vi "read_input_data.vi"(5 "Modulation info":T1={"Fs full"=0.0, "Fs high"=0.0, "Fs low"=0.0, "Read size"=5000, "FFT size low"=5000, "df low"=5000.0, "High carriers"=[], "Low carriers"=[], "Hi channels at low"=[7]} {"Hi channels at low" min=0 step=1; "Low carriers" format="%#_6p"; "High carriers" format="%#_6p"}, 7 "Config":T2={"IO params"={"Conversion"={"Rate"=4.0, "Num cards"=2, "Out channels"=4}, "Carriers"={"Phase shift"=180.0, "Levels"=[[0.8, 0.8, 0.8], [0.03, 0.03, 0.03]], "Delay samples"=73.15}, "TCP"={"Host"="192.168.1.15", "Port"=6666, "Buffering"=6, "Timeout"=6}, "Input channel sign"=[1, 1, 1]}, "High rate STFT"={"Win param"=101.5, "Window type"=61, "Win order"=2, "DFT size"=64, "Channels"=[7], "Oversample"=64}, "Low rate STFT"={"Win param"=120.0, "Window type"=61, "Win order"=8, "DFT size"=64, "Channels"=[7], "Oversample"=64}, "Filtering "=[]} {"Filtering"."Distortion"."Limit" format="%#_3p"; "Filtering"."Distortion"."LF cut" format="%#_3p"; "Filtering"."Kalman"."Measure noise" format="%#_3p"; "Filtering"."Kalman"."Process noise" format="%#_3p"; "Filtering"."Hum"."Limit" format="%#_3p"; "Filtering"."Hum"."Frequency" format="%#_4p"; "Low rate STFT"."Oversample" min=1 step=1; "Low rate STFT"."Channels" min=0 step=1; "Low rate STFT"."DFT size" min=1 step=1; "Low rate STFT"."Window type" items=["Rectangle"=0, "Hanning"=1, "Hamming"=2, "Blackman-Harris"=3, "Exact Blackman"=4, "Blackman"=5, "Flat Top"=6, "4 Term B-Harris "=7, "7 Term B-Harris"=8, "Low Sidelobe"=9, "Blackman Nuttall"=11, "Triangle"=30, "Bartlett-Hanning"=31, "Bohman"=32, "Parzen"=33, "Welch"=34, "Kaiser"=60, "Dolph-Chebyshev"=61, "Gaussian"=62]; "High rate STFT"."Oversample" min=1 step=1; "High rate STFT"."Channels" min=0 step=1; "High rate STFT"."DFT size" min=1 step=1; "High rate STFT"."Window type" items=["Rectangle"=0, "Hanning"=1, "Hamming"=2, "Blackman-Harris"=3, "Exact Blackman"=4, "Blackman"=5, "Flat Top"=6, "4 Term B-Harris "=7, "7 Term B-Harris"=8, "Low Sidelobe"=9, "Blackman Nuttall"=11, "Triangle"=30, "Bartlett-Hanning"=31, "Bohman"=32, "Parzen"=33, "Welch"=34, "Kaiser"=60, "Dolph-Chebyshev"=61, "Gaussian"=62]; "IO params"."Input channel sign" min=-1 max=1 step=1; "IO params"."Carriers"."Levels" min=0.0 step=0.1; "IO params"."Conversion"."Rate" format="%#_8g"}, 8 "error in":errorcluster, 11 "Connection in":refnum<k5>) -> (0 "error out":errorcluster, 1 "Restart IO":bool, 2 "Input data":waveform(dbl)[][](array[waveform]), 3 "Connection out":refnum<k5>, 4 "Sequence":u8)   [LabVIEW 2026]
uses:
  processing/ilemt_config.ctl
  IO_params.ctl
  processing/stft_params.ctl
  <vilib>/Analysis/4window.llb/windowTd.ctl
  processing/filter_params.ctl
  processing/detrend_mode.ctl
  processing/modulation_info.ctl
  <vilib>/Analysis/NI_AALPro.lvlib
panel:
  out "IO error":i32
  out "Sync error":i32
  out "length":i32
  in  "Timeouts":i32
  out "error IO":errorcluster
  # "Waveforms are scaled to range 0..1, rows are input cards and columns are XYZ channels."
  # "Read the input data using TCP"
  # "There was an error so we should restart IO"
  # "Locals:"
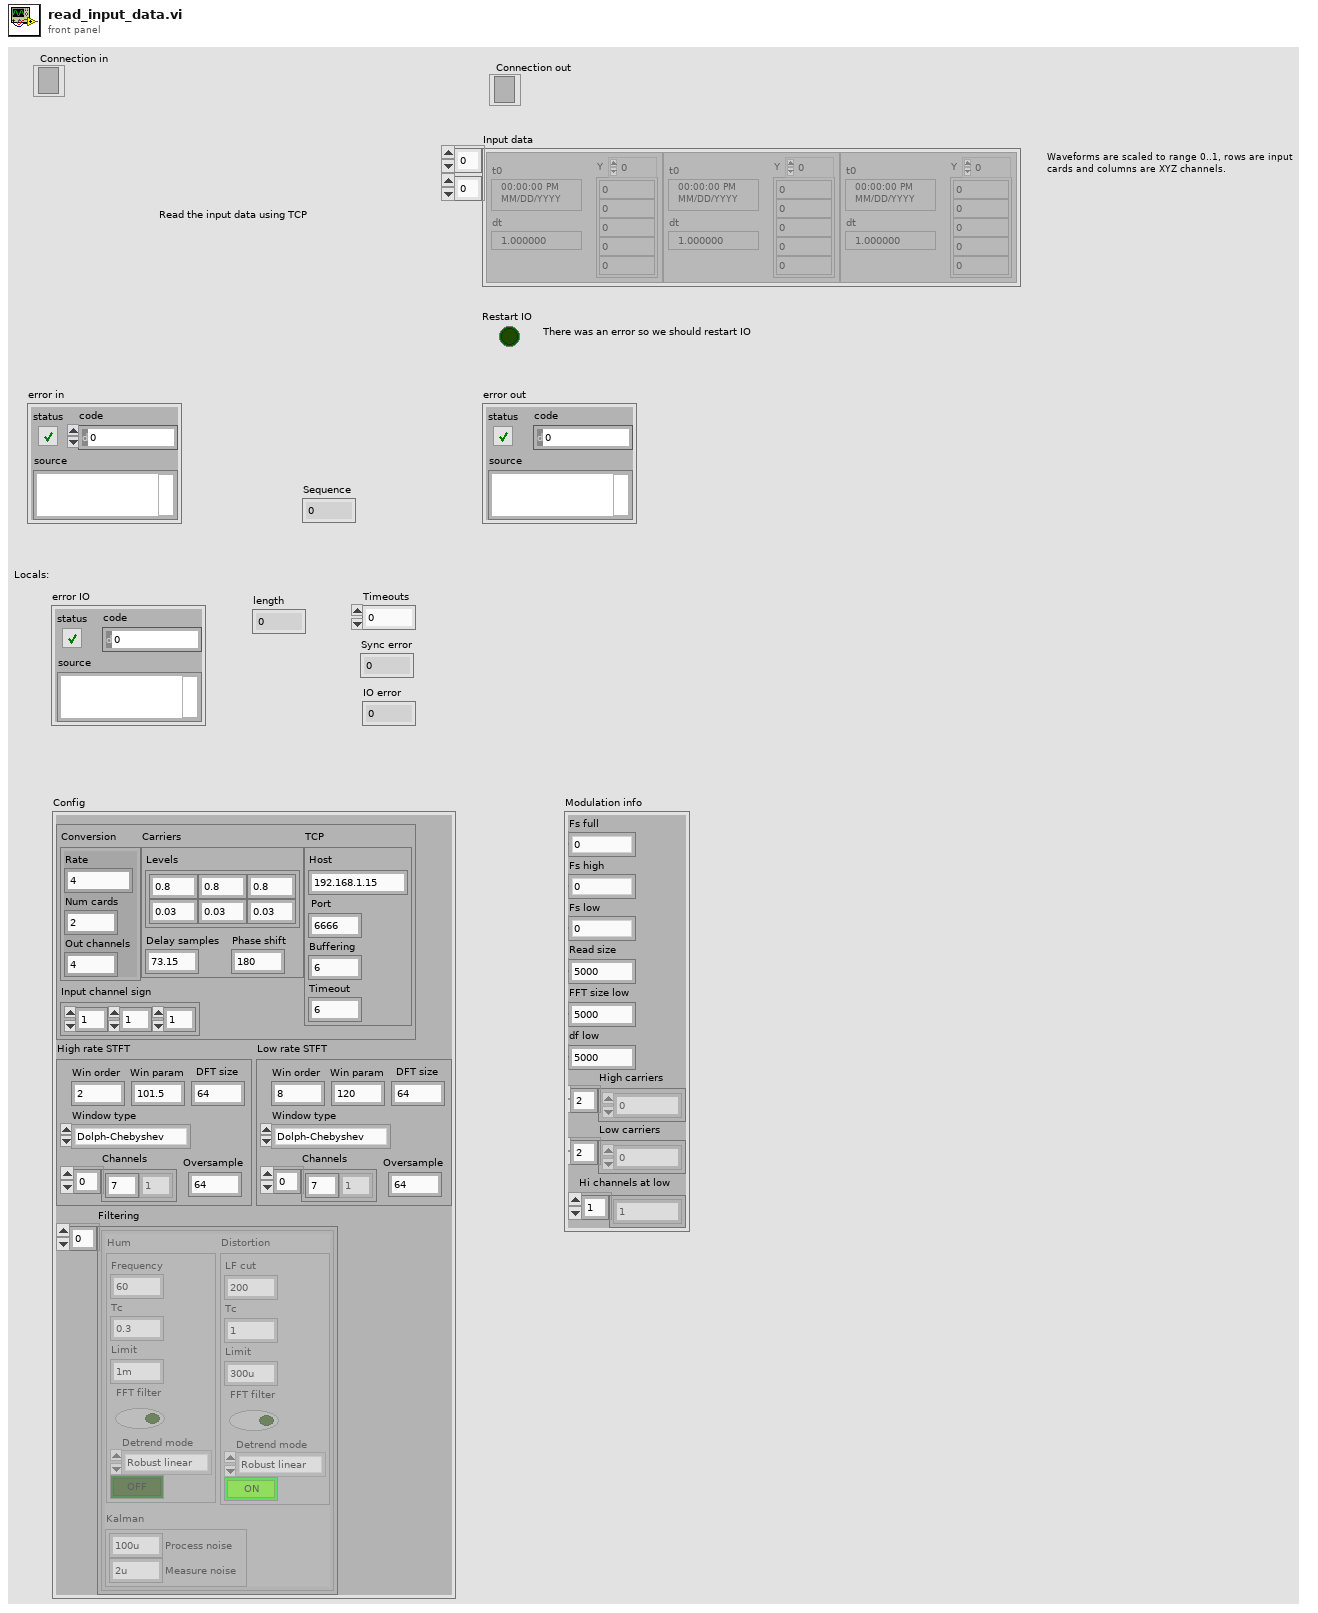
[diagram p1: front panel]
types:
  T1 = typedef "modulation_info.ctl" = cluster{"Fs full":dbl, "Fs high":dbl, "Fs low":dbl, "Read size":i32, "FFT size low":i32, "df low":dbl, "High carriers":dbl[], "Low carriers":dbl[], "Hi channels at low":i32[]}
  T2 = typedef "ilemt_config.ctl" = cluster{"IO params":T3, "High rate STFT":T4, "Low rate STFT":T4, "Filtering ":T6[]}
  T3 = typedef "IO_params.ctl" = cluster{"Conversion":cluster{"Rate":dbl, "Num cards":u32, "Out channels":u32}, "Carriers":cluster{"Phase shift":dbl, "Levels":dbl[][], "Delay samples":dbl}, "TCP":cluster{"Host":string, "Port":i32, "Buffering":u32, "Timeout":u32}, "Input channel sign":i32[]}
  T4 = typedef "stft_params.ctl" = cluster{"Win param":dbl, "Window type":T5, "Win order":i32, "DFT size":i32, "Channels":i32[], "Oversample":i32}
  T5 = typedef "NI_AALPro.lvlib/windowTd.ctl" = u32
  T6 = typedef "filter_params.ctl" = cluster{"Hum":cluster{"Frequency":dbl, "Tc":dbl, "Limit":dbl, "FFT filter":bool, "Detrend mode":T7, "Enable":bool}, "Kalman":cluster{"Process noise":dbl, "Measure noise":dbl}, "Distortion":cluster{"LF cut":dbl, "Tc":dbl, "Limit":dbl, "FFT filter":bool, "Detrend mode":T7, "Enable":bool}}
  T7 = typedef "detrend_mode.ctl" = enum16{"Zero mean", "Linear", "Robust linear"}
  T8 = enum16{"Standard", "Buffered", "CRLF", "Immediate"}
  T9 = enum16{"big-endian, network order", "native, host order", "little-endian"}
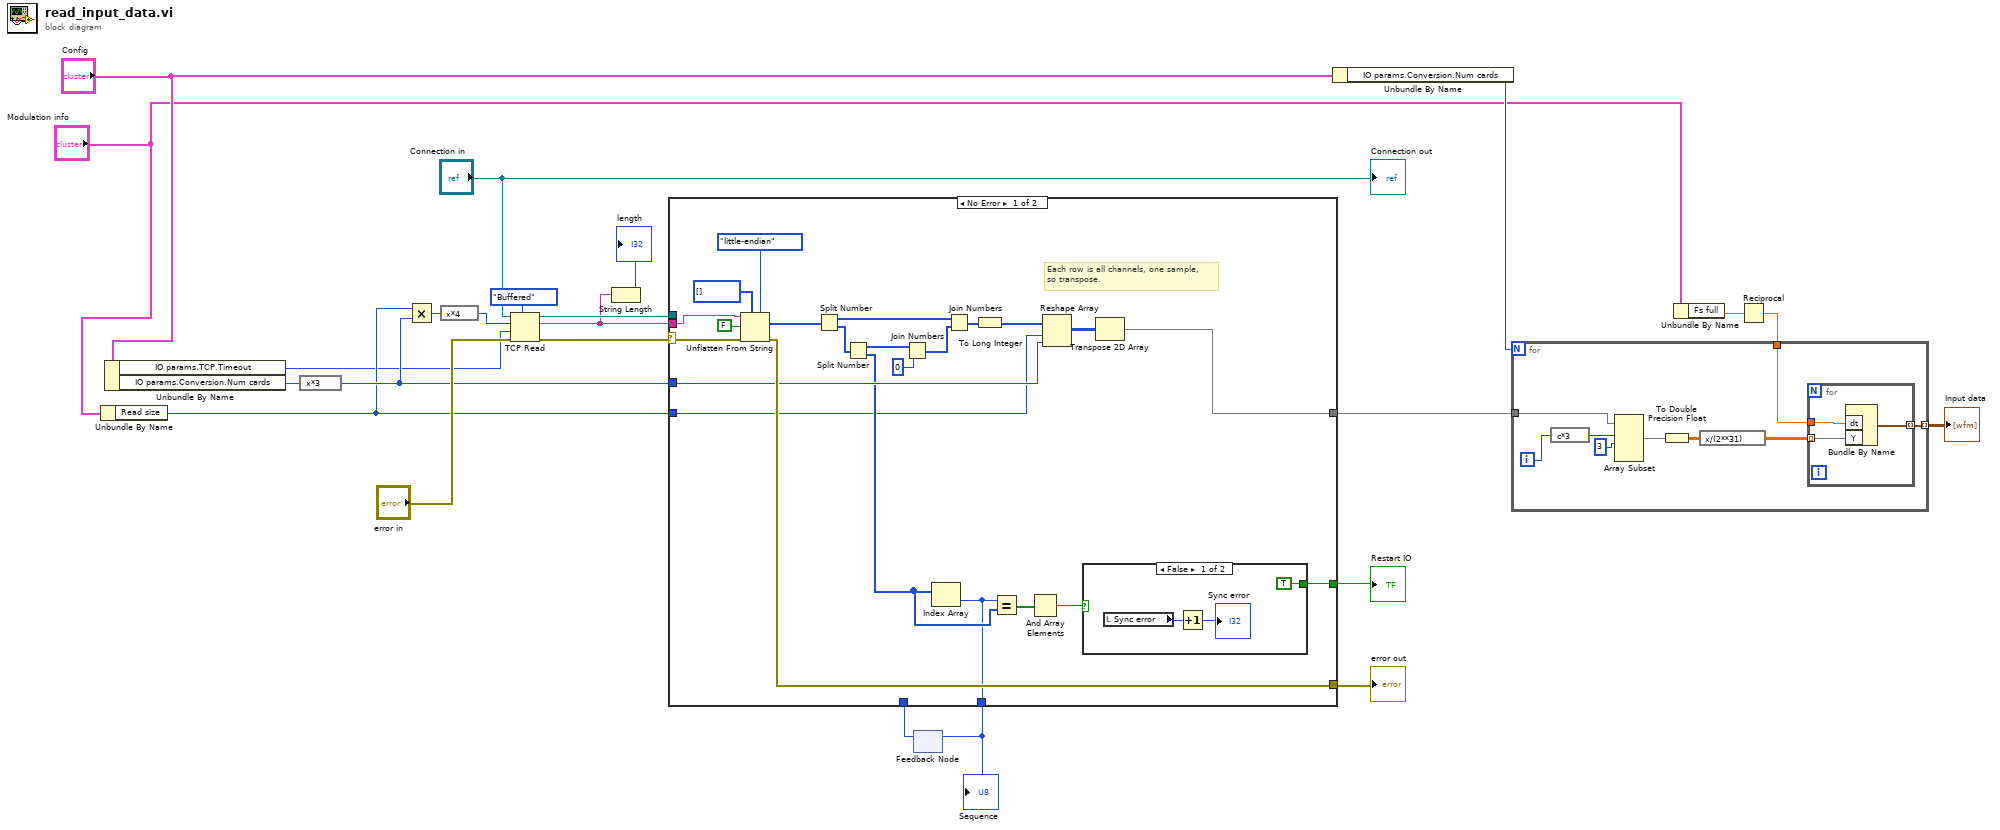
[diagram p0: block diagram]
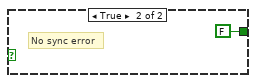
[diagram p2: hidden frame]
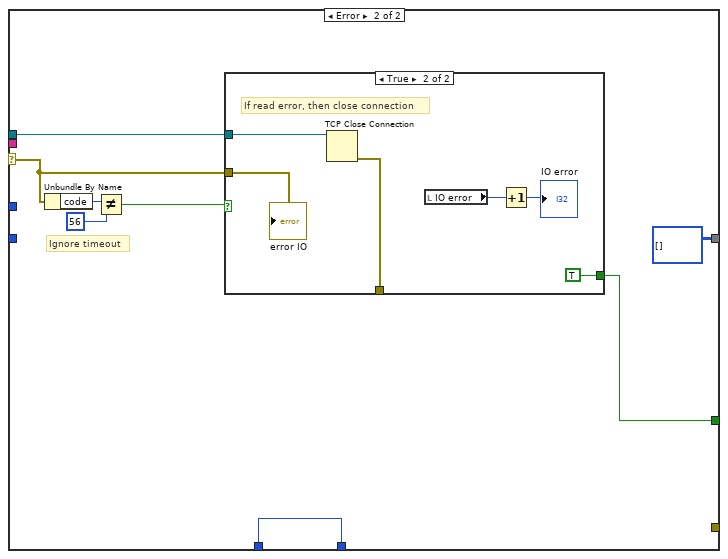
[diagram p3: hidden frame]
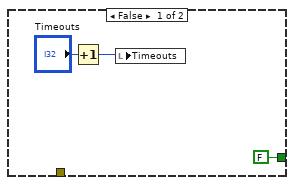
[diagram p4: hidden frame]
diagram:
  n1 = Unbundle By Name("Modulation info") -> ("Read size"=w4:i32)
  n2 = Unbundle By Name("Config") -> ("IO params.TCP.Timeout"=w3:u32, "IO params.Conversion.Num cards"=w8:u32)
  n3 = expression code="x*3"(w8) -> (w22:u32)
  n4 = Multiply(x=w4, y=w22) -> (x*y=w12:u32)
  n5 = expression code="x*4"(w12) -> (w11:u32)
  n6 = TCP Read(connection ID="Connection in", bytes to read=w11, error in (no error)="error in", 7:T8."Buffered" ("mode (standard)"), 9:w3) -> (connection ID out=w13:refnum<k5>, data out=w9:string, error out=w14:errorcluster)
  n7 = String Length(string=w9) -> (length=→"length":i32)
  n8 = feedback #1() -> (w1:u8)  [unwired: 1 in]
  n9 = case shown="No Error" w14 {
    selector: w14 -> [w45 w58]
    tunnel: [w29 i32[][] []] -> w21
    tunnel: [w47 _] -> w24
    tunnel: w9 -> [w46 _]
    tunnel: w13 -> [_ w59]
    tunnel: w22 -> [w41 _]
    tunnel: [w31 w54] -> w16
    tunnel: w4 -> [w30 _]
    tunnel: [w25 w52] -> w2
    tunnel: w1 -> [_ w52]
    frame No Error {
      # "Each row is all channels, one sample,  so transpose."
      n10 = Unflatten From String(type=i32[] [] ("size(s)"), binary string=w46, data includes array or string size? (T)=FALSE, byte order (0:big-endian, network order)=T9."little-endian", error in (no error)=w45) -> (value=w32:i32[], error out=w47:errorcluster)  [unwired: 1 out]
      n11 = Split Number(x=w32) -> (hi(x)=w38:u16[], lo(x)=w39:u16[])
      n12 = Split Number(x=w39) -> (hi(x)=w36:u8[], lo(x)=w34:u8[])
      n13 = Join Numbers(hi=w36, lo=u8 0 ("index")) -> ((hi.lo)=w37:u16[])
      n14 = Index Array(array=w34) -> (element=w25:u8)  [unwired: 1 in]
      n15 = Join Numbers(hi=w38, lo=w37) -> ((hi.lo)=w28:u32[])
      n16 = To Long Integer(number=w28) -> (32bit integer=w27:i32[])
      n17 = Equal?(x=w25, y=w34) -> (x = y?=w33:bool[])
      n18 = And Array Elements(Boolean array=w33) -> (logical AND=w26:bool)
      n19 = Reshape Array(w27, w30, w41) -> (w40:i32[][])
      n20 = case shown="False" w26 {
        tunnel: [TRUE ("x != y?") FALSE ("x != y?")] -> w31
        frame False {
          n21 = local read "Sync error"() -> (w50:i32)
          n22 = Increment(x=w50) -> (x+1=→"Sync error":i32)
        }
        frame True {
          # "No sync error"
        }
      }
      n23 = Transpose 2D Array(2D array=w40) -> (transposed array=w29:i32[][])
    }
    frame Error {
      # "Ignore timeout"
      n24 = Unbundle By Name(w58) -> ("code"=w57:i32)
      n25 = Not Equal?(x=w57, y=56) -> (x != y?=w55:bool)
      n26 = case shown="True" w55 {
        tunnel: w59 -> [_ w68]
        tunnel: [_ w67] -> _
        tunnel: w58 -> [_ w66]
        tunnel: [FALSE ("x != y?") TRUE ("x != y?")] -> w54
        frame False {
          n27 = Increment(x="Timeouts") -> (x+1=w61:i32)
          n28 = local write "Timeouts"(w61) -> ()
        }
        frame True {
          # "If read error, then close connection"
          n29 = TCP Close Connection(connection ID=w68) -> (error out=w67:errorcluster)  [unwired: 2 in, 1 out]
          n30 = local read "IO error"() -> (w65:i32)
          n31 = Increment(x=w65) -> (x+1=→"IO error":i32)
          "error IO" <- w66
        }
      }
    }
  }
  "error out" <- w24
  "Restart IO" <- w16
  "Sequence" <- w2
  n32 = feedback-in #1(w2) -> ()
  n33 = Unbundle By Name("Config") -> ("IO params.Conversion.Num cards"=w20:u32)
  n34 = Unbundle By Name("Modulation info") -> ("Fs full"=w19:dbl)
  n35 = Reciprocal(x=w19) -> (1/x=w18:dbl)
  n36 = for {
    N: w20 -> [_]
    tunnel: w21 -> [w77]
    tunnel: [w72] -> w17 mode=indexing
    tunnel: w18 -> [w69]
    i -> [w74]
    n37 = expression code="c*3"(w74) -> (w76:i32)
    n38 = Array Subset(array=w77, index (row)=w76, length (row)=3 ("length")) -> (w73:i32[][])  [unwired: 2 in]
    n39 = To Double Precision Float(number=w73) -> (double precision float=w71:dbl[][])
    n40 = expression code="x/(2**31)"(w71) -> (w70:dbl[][])
    n41 = for {
      tunnel: w70 -> [w80] mode=indexing
      tunnel: [w79] -> w72 mode=indexing
      tunnel: w69 -> [w78]
      n42 = Bundle By Name("dt"=w78, "Y"=w80) -> (w79:waveform(dbl))  [unwired: 1 in]
    }
  }
  "Input data" <- w17
  "Connection out" <- "Connection in"
